vi "Rcv Cmd.vi"(8 "error in":errorcluster, 11 "cCRDS in":refnum<class "cCRDS.lvclass">=refnum) -> (0 "error out":errorcluster, 3 "cCRDS out":refnum<class "cCRDS.lvclass">)   [LabVIEW 2015, in "cCRDS.lvclass"]
uses:
  cCRDS.lvclass
  cCRDS.lvclass/cCRDS.ctl
  Reusable/Instrument/state.ctl
  <vilib>/DAQmx/write.llb/DAQmx Write (Digital 1D Bool NChan 1Samp 1Line).vi
  Reusable/CRDS/Main/Write writeRDs.vi
  <vilib>/DAQmx/miscellaneous.llb/DAQmx Fill In Error Info.vi
  Reusable/Instrument/Instrument.lvclass
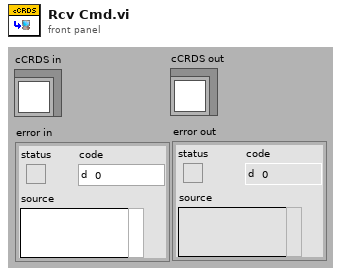
[diagram p1: front panel]
types:
  T1 = typedef "Instrument.lvclass/state.ctl" = enum8{"Configure", "Acquire", "Wait", "Quit", "Handle Error", "NOOP"}
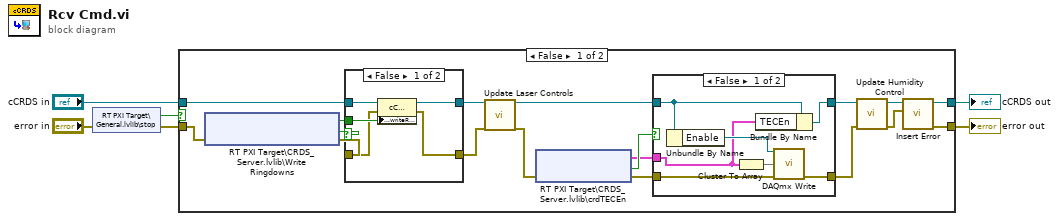
[diagram p0: block diagram]
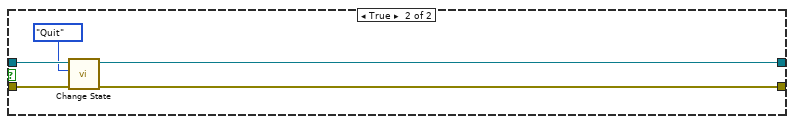
[diagram p4: hidden frame]
diagram:
  n1 = shared-variable "RT PXI Target\\General.lvlib\\stop"(error in="error in") -> (w4:bool, error out=w3:errorcluster)
  n2 = case shown="False" w4 {
    tunnel: [w18 w42] -> w6
    tunnel: "cCRDS in" -> [w15 w44]
    tunnel: [w24 w45] -> w1
    tunnel: w3 -> [w13 w43]
    frame False {
      n3 = shared-variable "RT PXI Target\\CRDS_Server.lvlib\\Write Ringdowns"(error in=w13) -> (w8:bool, error out=w7:errorcluster, w9:bool)  [unwired: 1 in]
      n4 = case shown="False" w9 {
        tunnel: w15 -> [w25 w31]
        tunnel: [w29 w31] -> w14
        tunnel: w8 -> [w28 _]
        tunnel: w7 -> [w27 w30]
        tunnel: [w26 w30] -> w12
        frame False {
          n5 = property class="cCRDS"(reference=w25, error in=w27, "Accessors:writeRDs"=w28) -> (reference out=w29:refnum<class "cCRDS.lvclass">, error out=w26:errorcluster)
        }
        frame True {
        }
      }
      n6 = call "Update Laser Controls.vi"("cCRDS in"=w14, "error in"=w12) -> ("cCRDS out"=w17:refnum<class "cCRDS.lvclass">, "error out"=w11:errorcluster)  [unwired: 16 in]
      n7 = shared-variable "RT PXI Target\\CRDS_Server.lvlib\\crdTECEn"(error in=w11) -> (w22:cluster{"med":bool, "high":bool}, error out=w21:errorcluster, w23:bool)  [unwired: 1 in]
      n8 = case shown="False" w23 {
        tunnel: w22 -> [w34 _]
        tunnel: w21 -> [w37 w40]
        tunnel: [w36 w40] -> w10
        tunnel: w17 -> [w32 w39]
        tunnel: [w33 w39] -> w16
        frame False {
          n9 = Unbundle By Name(w32) -> ("Enable"=w35:refnum<k21>)
          n10 = Cluster To Array(cluster=w34) -> (array=w38:bool[])
          n11 = Bundle By Name(cluster=w32, "TECEn"=w34) -> (w33:refnum<class "cCRDS.lvclass">)
          n12 = call-poly <vilib>:"DAQmx Write.vi"("task/channels in"=w35, "data"=w38, "error in"=w37) -> ("error out"=w36:errorcluster)  [unwired: 10 in, 2 out]
        }
        frame True {
        }
      }
      n13 = call "Update Humidity Control.vi"("error in"=w10, "cCRDS in"=w16) -> ("error out"=w20:errorcluster, "cCRDS out"=w19:refnum<class "cCRDS.lvclass">)  [unwired: 8 in]
      n14 = call "Insert Error.vi"("err"=w20, "Instrument in"=w19) -> ("error out"=w18:errorcluster, "Instrument out"=w24:refnum<class "cCRDS.lvclass">)  [unwired: 7 in, 1 out]
    }
    frame True {
      n15 = call "Change State.vi"("error in"=w43, "instr state"=state."Quit", "Instrument in"=w44) -> ("error out"=w42:errorcluster, "Instrument out"=w45:refnum<class "cCRDS.lvclass">)  [unwired: 7 in]
    }
  }
  "error out" <- w6
  "cCRDS out" <- w1
